vi "웹서버 데이터 쓰기.vi"(8 "에러 입력(에러 없음)":errorcluster, 10 "클러스터":cluster{"0":string}, 11 "참조 번호 입력":T1 caption="client handle out") -> (0 "error out":errorcluster caption="에러 출력", 1 "body 3":string caption="웹서버에 입력된 문자열", 2 "headers 3":string caption="연결확인 메세지 출력", 3 "참조 번호 출력":T1 caption="client handle out")   [LabVIEW 2019]
uses:
  <vilib>/httpClient/ClientHandle.ctl
  <vilib>/httpClient/PUTBuffer.vi
  <vilib>/httpClient/LabVIEWHTTPClient.lvlib
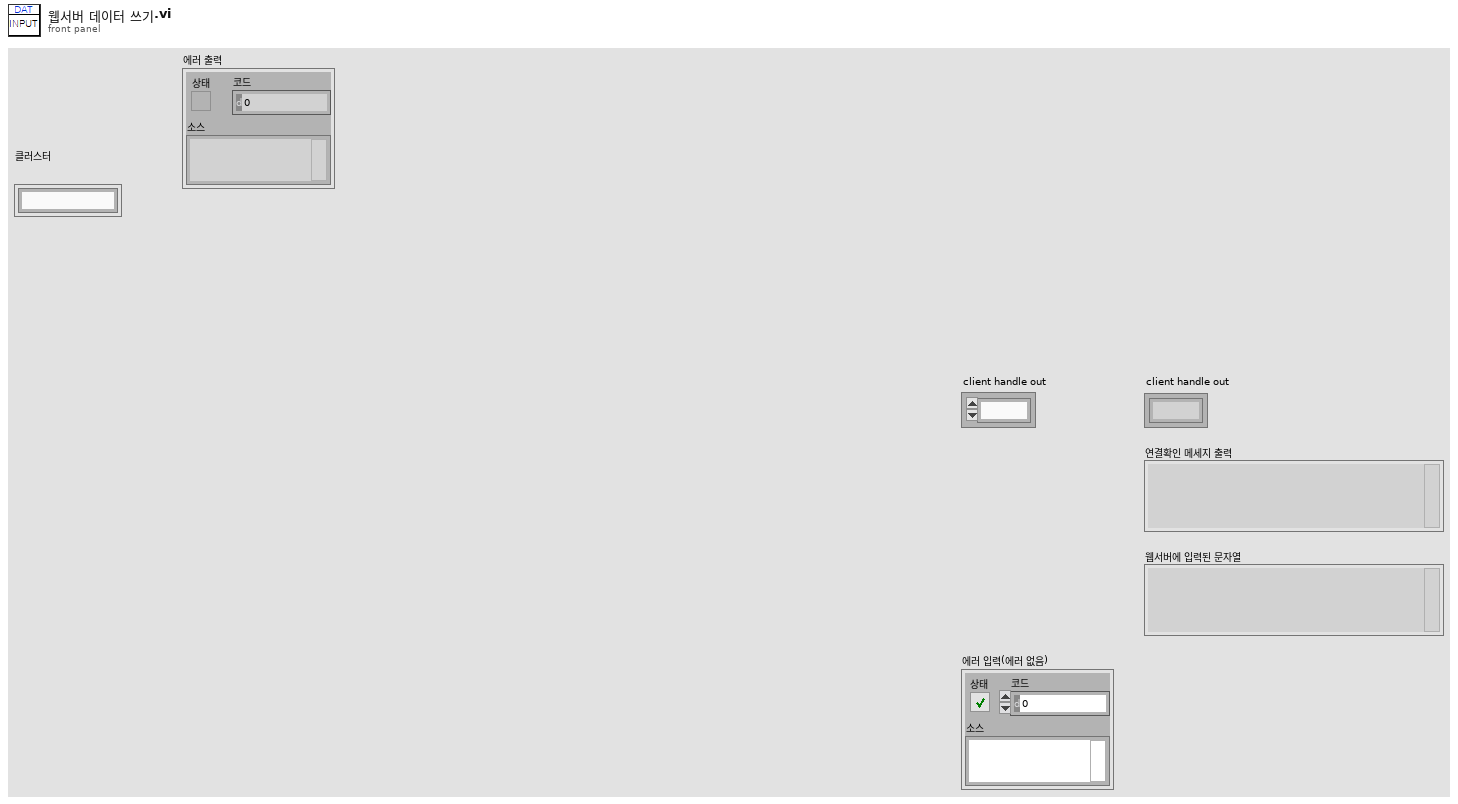
[diagram p1: front panel]
types:
  T1 = typedef "LabVIEWHTTPClient.lvlib/ClientHandle.ctl" = refnum<k1>
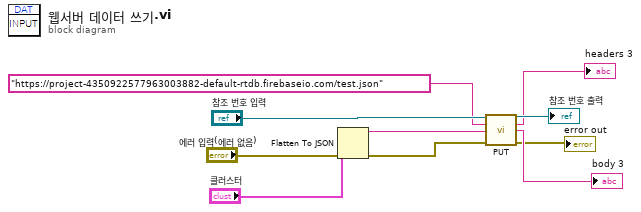
[diagram p0: block diagram]
diagram:
  n1 = Flatten To JSON(anything="클러스터", error in (no error)="에러 입력(에러 없음)") -> (JSON string=w4:string, 11:w3:errorcluster)  [unwired: 1 in]
  n2 = call-poly <vilib>:"PUT.vi"("client handle"="참조 번호 입력", "url"="https://project-4350922577963003882-default-rtdb.firebaseio.com/test.json", "buffer"=w4, "error in (no error)"=w3) -> ("client handle out"=→"참조 번호 출력":T1, "headers"=→"headers 3":string, "body"=→"body 3":string, "error out"=→"error out":errorcluster)  [unwired: 8 in]
